vi "HandleAlarms.vi"(8 "error in (no error)":errorcluster, 11 "NeedleValve in":refnum<class "NeedleValve.lvclass">) -> (0 "error out":errorcluster, 3 "NeedleValve out":refnum<class "NeedleValve.lvclass">)   [LabVIEW 2019, in "NeedleValve.lvclass"]
uses:
  NeedleValve.lvclass
  NeedleValve.lvclass/NeedleValve.ctl
  modbus engine custom/MB_MODULE_class/MB_MODULE.lvclass/MB_MODULE.ctl
  DA_class/DA.lvclass/DA.ctl
  Proccess_class/Proccess.lvclass/Proccess.ctl
  subvis/bool_change.vi
  DA_class/private/write_to_db.vi
  Proccess_class/GetNames.vi
  Proccess_class/GetLogger.vi
  modbus engine custom/MB_ENGINE_class/MB_ENGINE.lvclass
  C:/Users/ANENKOV_V1/Desktop/src/modbus engine custom/MB_MODULE_class/MB_MODULE.lvclass
  DA_class/DA.lvclass
  C:/Users/ANENKOV_V1/Desktop/src/Proccess_class/Proccess.lvclass
  Logger_class/WriteEvent.vi
  modbus engine custom/MB_MODULE_class/MB_MODULE.lvclass
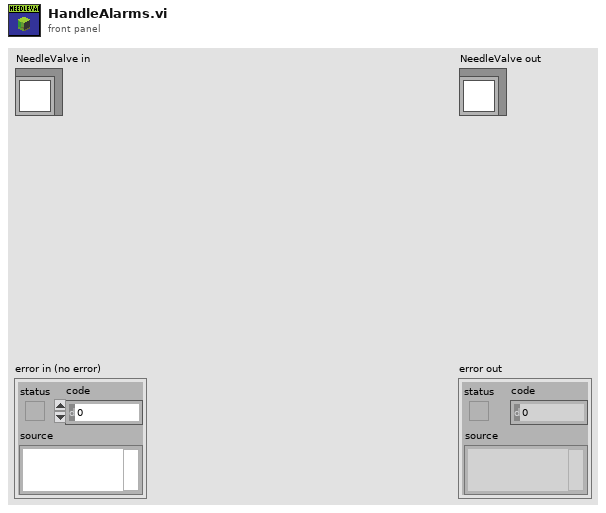
[diagram p1: front panel]
types:
  T1 = typedef "Needle Valve Data.ctl" = cluster{"Engine State":T2, "StateValveModbus":T3, "Alarms":T4, "RAW":i32, "Angele":dbl, "Step":i32, "Encoder":i32, "Kinematic":T5, "Limits":T6, "EncoderMax":i32, "Counter Max Dont Update":i32, "EncoderMin":i32, "Counter Min Dont Update":i32, "Prepere Counter":i32, "STEP INIT":i32, "offset - Angel":dbl}
  T2 = typedef "MB_ENGINE.lvclass/Engine State.ctl" = u16
  T3 = typedef "Needle Valve State.ctl" = enum16{"STOPED", "CLOSED", "OPENED", "OPENING", "CLOSING", "FULL_CLOSE"}
  T4 = typedef "MB_ENGINE.lvclass/Engine Alarms.ctl" = cluster{"OL":bool, "TF":bool, "STL":bool, "OCP":bool, "CPUV":bool, "UVLO":bool, "SPI_ERROR":bool, "Fault":bool, "OL 2":bool, "TF 2":bool, "STL 2":bool, "OCP 2":bool, "CPUV 2":bool, "UVLO 2":bool, "reserved":bool, "InitDone":bool}
  T5 = typedef "MB_ENGINE.lvclass/Settings.ctl" = cluster{"ACC Steps Per Sec^2":u16, "DEC Steps Per Sec^2":u16, "Min Velosity Step Per Sec":u16, "Max Velosity Step Per Sec":u16, "MicroStep":u16}
  T6 = typedef "MB_ENGINE.lvclass/Limits Status.ctl" = cluster{"Fault 2 Switch":bool, "Fault 1 Switch":bool, "Center(Home)":bool, "Lower Limit":bool, "Upper Limit":bool}
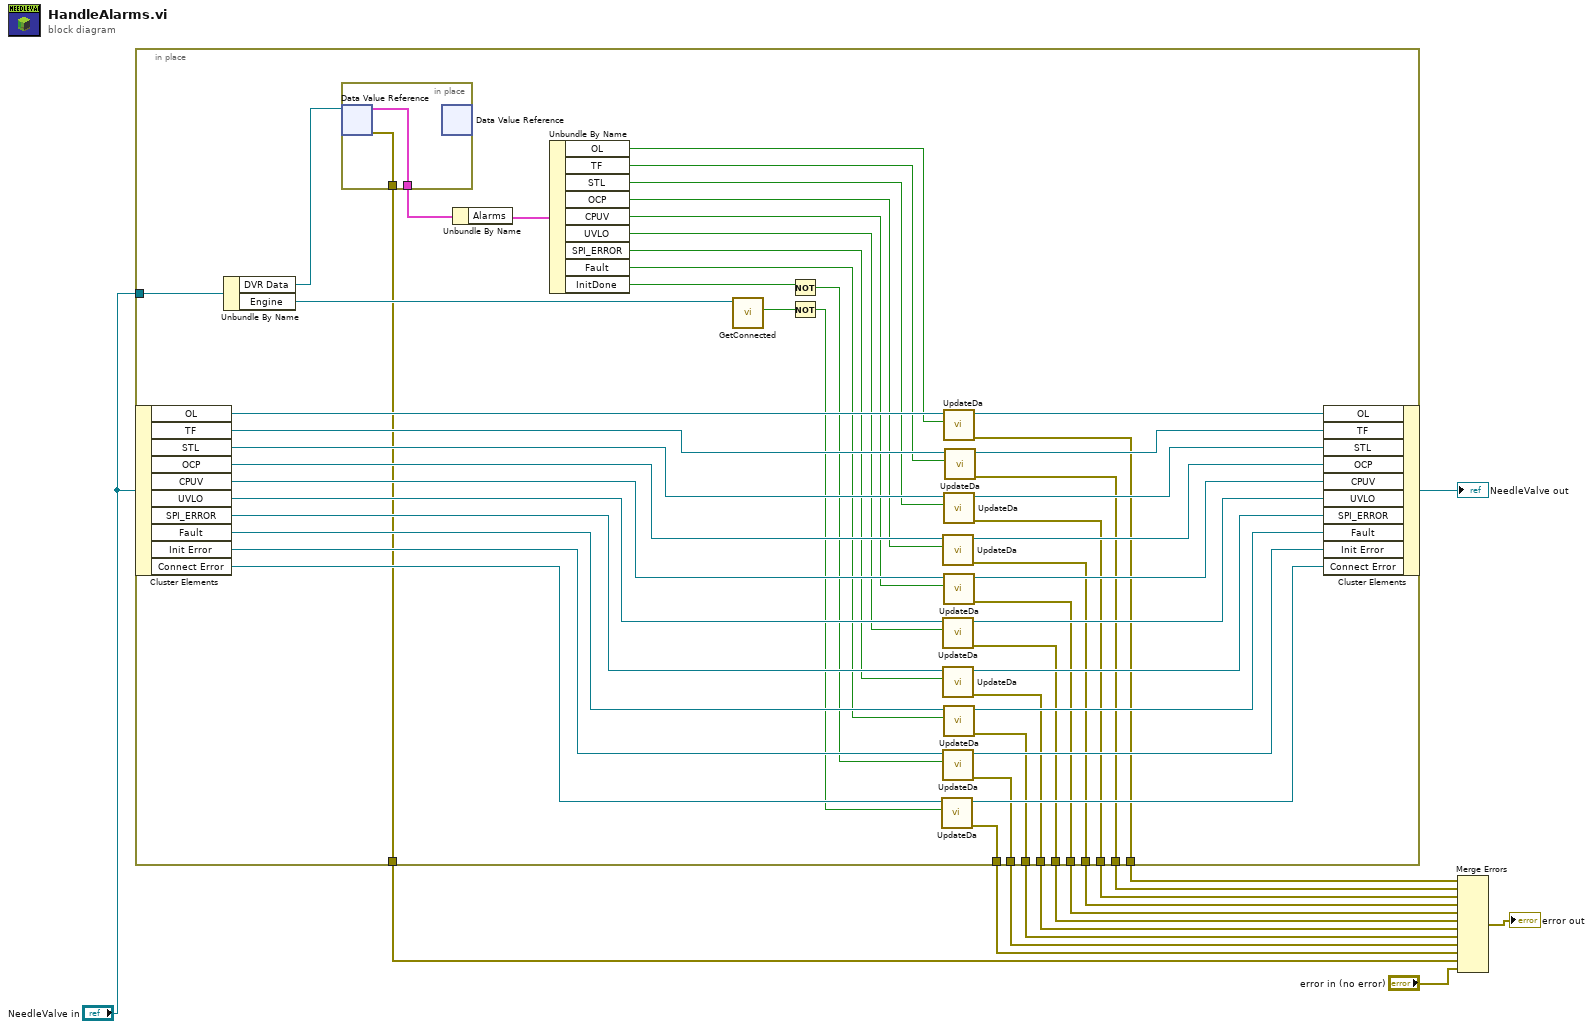
[diagram p0: block diagram]
diagram:
  n1 = in-place {
    in-place-border: [w43] -> w5
    in-place-border: [w42] -> w6
    in-place-border: [w41] -> w7
    in-place-border: [w40] -> w8
    in-place-border: [w39] -> w9
    in-place-border: [w38] -> w10
    in-place-border: [w37] -> w11
    in-place-border: [w36] -> w12
    in-place-border: [w35] -> w13
    in-place-border: [w34] -> w14
    in-place-border: "NeedleValve in" -> [w21]
    in-place-border: [w16] -> w1
    n2 = in-place-cluster #1("NeedleValve in") -> ("OL"=w63:refnum<class "DA.lvclass">, "TF"=w61:refnum<class "DA.lvclass">, "STL"=w60:refnum<class "DA.lvclass">, "OCP"=w59:refnum<class "DA.lvclass">, "CPUV"=w58:refnum<class "DA.lvclass">, "UVLO"=w57:refnum<class "DA.lvclass">, "SPI_ERROR"=w56:refnum<class "DA.lvclass">, "Fault"=w55:refnum<class "DA.lvclass">, "Init Error"=w54:refnum<class "DA.lvclass">, "Connect Error"=w53:refnum<class "DA.lvclass">)
    n3 = Unbundle By Name(w21) -> ("DVR Data"=w19:refnum<data-value>, "Engine"=w20:refnum<class "MB_ENGINE.lvclass">)
    n4 = in-place {
      in-place-border: [w65] -> w18
      in-place-border: [w64] -> w16
      n5 = in-place-dvr #2(w19) -> (w65:T1, w64:errorcluster)
      n6 = in-place-dvr #2() -> ()  [unwired: 1 in, 2 out]
    }
    n7 = Unbundle By Name(w18) -> ("Alarms"=w17:T4)
    n8 = Unbundle By Name(w17) -> ("OL"=w33:bool, "TF"=w32:bool, "STL"=w31:bool, "OCP"=w30:bool, "CPUV"=w29:bool, "UVLO"=w28:bool, "SPI_ERROR"=w27:bool, "Fault"=w26:bool, "InitDone"=w25:bool)
    n9 = call "GetConnected.vi"("MB_MODULE in"=w20) -> ("Connected"=w23:bool)  [unwired: 10 in]
    n10 = Not(x=w25) -> (.not. x?=w24:bool)
    n11 = Not(x=w23) -> (.not. x?=w22:bool)
    n12 = call "UpdateDa.vi"("RAW"=w22, "Sig_DA in"=w53) -> ("error out"=w43:errorcluster, "Sig_DA out"=w44:refnum<class "DA.lvclass">)  [unwired: 7 in, 1 out]
    n13 = call "UpdateDa.vi"("RAW"=w30, "Sig_DA in"=w59) -> ("error out"=w37:errorcluster, "Sig_DA out"=w50:refnum<class "DA.lvclass">)  [unwired: 7 in, 1 out]
    n14 = call "UpdateDa.vi"("RAW"=w28, "Sig_DA in"=w57) -> ("error out"=w39:errorcluster, "Sig_DA out"=w48:refnum<class "DA.lvclass">)  [unwired: 7 in, 1 out]
    n15 = call "UpdateDa.vi"("RAW"=w27, "Sig_DA in"=w56) -> ("error out"=w40:errorcluster, "Sig_DA out"=w47:refnum<class "DA.lvclass">)  [unwired: 7 in, 1 out]
    n16 = call "UpdateDa.vi"("RAW"=w24, "Sig_DA in"=w54) -> ("error out"=w42:errorcluster, "Sig_DA out"=w45:refnum<class "DA.lvclass">)  [unwired: 7 in, 1 out]
    n17 = call "UpdateDa.vi"("RAW"=w33, "Sig_DA in"=w63) -> ("error out"=w34:errorcluster, "Sig_DA out"=w62:refnum<class "DA.lvclass">)  [unwired: 7 in, 1 out]
    n18 = call "UpdateDa.vi"("RAW"=w31, "Sig_DA in"=w60) -> ("error out"=w36:errorcluster, "Sig_DA out"=w51:refnum<class "DA.lvclass">)  [unwired: 7 in, 1 out]
    n19 = call "UpdateDa.vi"("RAW"=w29, "Sig_DA in"=w58) -> ("error out"=w38:errorcluster, "Sig_DA out"=w49:refnum<class "DA.lvclass">)  [unwired: 7 in, 1 out]
    n20 = call "UpdateDa.vi"("RAW"=w26, "Sig_DA in"=w55) -> ("error out"=w41:errorcluster, "Sig_DA out"=w46:refnum<class "DA.lvclass">)  [unwired: 7 in, 1 out]
    n21 = call "UpdateDa.vi"("RAW"=w32, "Sig_DA in"=w61) -> ("error out"=w35:errorcluster, "Sig_DA out"=w52:refnum<class "DA.lvclass">)  [unwired: 7 in, 1 out]
    n22 = in-place-cluster #1("OL"=w62, "TF"=w52, "STL"=w51, "OCP"=w50, "CPUV"=w49, "UVLO"=w48, "SPI_ERROR"=w47, "Fault"=w46, "Init Error"=w45, "Connect Error"=w44) -> (→"NeedleValve out":refnum<class "NeedleValve.lvclass">)
  }
  n23 = Merge Errors(w14, w13, w12, w11, w10, w9, w8, w7, w6, w5, w1, "error in (no error)") -> (→"error out":errorcluster)
